vi "Peak.vi"(11 "TypedCircularBuffer in":refnum<class "RefTypedCircularBuffer.lvclass">) -> (1 "invalid?":bool, 2 "element":T1, 3 "TypedCircularBuffer out":refnum<class "RefTypedCircularBuffer.lvclass">)   [LabVIEW 2024, in "RefTypedCircularBuffer.lvclass"]
uses:
  RefTypedCircularBuffer.lvclass
  Type.ctl
  RefTypedCircularBuffer.lvclass/RefTypedCircularBuffer.ctl
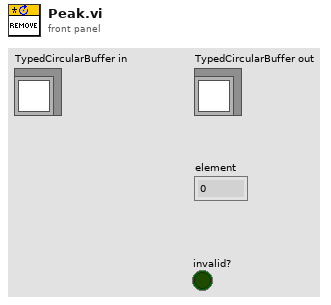
[diagram p1: front panel]
types:
  T1 = typedef "RefTypedCircularBuffer.lvclass/Type.ctl" = u8
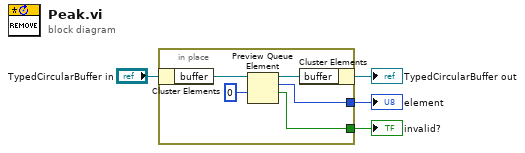
[diagram p0: block diagram]
diagram:
  n1 = in-place {
    in-place-border: [w5] -> w2
    in-place-border: [w6] -> w1
    n2 = in-place-cluster #1("TypedCircularBuffer in") -> ("buffer"=w9:refnum<queue>)
    n3 = Preview Queue Element(queue=w9, timeout in ms (-1)=0) -> (queue out=w8:refnum<queue>, element=w5:T1, timed out?=w6:bool)  [unwired: 1 in, 1 out]
    n4 = in-place-cluster #1("buffer"=w8) -> (→"TypedCircularBuffer out":refnum<class "RefTypedCircularBuffer.lvclass">)
  }
  "element" <- w2
  "invalid?" <- w1
